vi "Stream Split Character Match RegExp Std Out.vi"(8 "error in (no error)":errorcluster, 11 "Bad Regex in":refnum<class "Bad Regex.lvclass">) -> (0 "error out":errorcluster, 2 "Stream Split Character Match RegExp Std Out":string)   [LabVIEW 2020, in "ase.test.lvlib" / "Bad Regex.lvclass"]
uses:
  Bad Regex.lvclass
  Bad Regex.lvclass/Bad Regex.ctl
  ase/configuration/configuration.lvclass
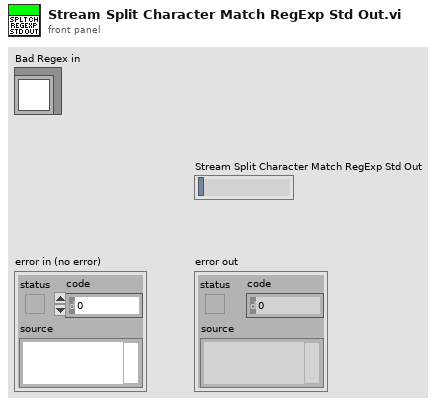
[diagram p1: front panel]
types:
  T1 = typedef "ase.test.lvlib/Bad Regex.lvclass/Bad Value.ctl" = enum16{"Out", "Err", "Both"}
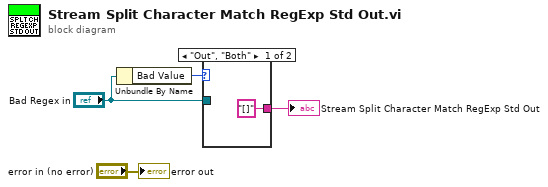
[diagram p0: block diagram]
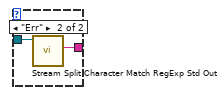
[diagram p2: hidden frame]
diagram:
  n1 = Unbundle By Name("Bad Regex in") -> ("Bad Value"=w3:T1)
  n2 = case shown="\"Out\", \"Both\"" w3 {
    tunnel: ["[]" w6] -> w2
    tunnel: "Bad Regex in" -> [_ w7]
    frame "Out", "Both" {
    }
    frame "Err" {
      n3 = call-parent "Stream Split Character Match RegExp Std Out.vi"("configuration in"=w7) -> ("Stream Split Character Match RegExp Std Out"=w6:string)  [unwired: 9 in, 1 out]
    }
  }
  "Stream Split Character Match RegExp Std Out" <- w2
  "error out" <- "error in (no error)"
